vi "9702 Mapping failed for index at sub-index--error.vi"(8 "error in (no error)":errorcluster, 10 "Sub-Index":u8 format="%.0x", 11 "Index":u16) -> (0 "error out":errorcluster)   [LabVIEW 2020, in "PDO Grid.lvlib"]
uses:
  EDS-File-Viewer/source/PDO Grid.lvlib
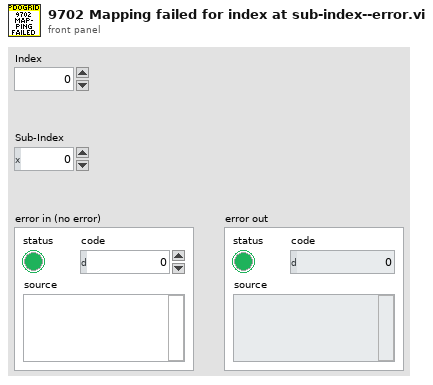
[diagram p1: front panel]
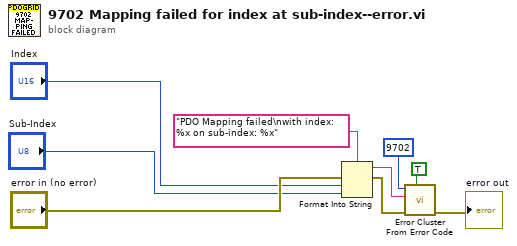
[diagram p0: block diagram]
diagram:
  n1 = Format Into String(format string="PDO Mapping failed\nwith index: %x on sub-index: %x", error in="error in (no error)", "Index", "Sub-Index") -> (resulting string=w4:string, error out=w8:errorcluster)  [unwired: 1 in]
  n2 = call <vilib>:"Error Cluster From Error Code.vi"("show call chain? (False)"=TRUE, "error in (no error)"=w8, "error message (\"\")"=w4, "error code (0)"=9702) -> ("error out"=→"error out":errorcluster)  [unwired: 5 in]
